vi "PHD2000 RUN SURE.vi"(8 "error in (no error)":errorcluster, 10 "Pump #":string, 11 "VISA resource name 2":refnum<visa-resource-name>) -> (0 "error out":errorcluster, 3 "VISA resource name out":refnum<visa-resource-name>)   [LabVIEW 2017]
uses:
  <instrlib>/Harvard Syringe Pump PHD2000/Harvard Syringe Pump PHD2000.lvlib
panel:
  out "Pump stop":bool
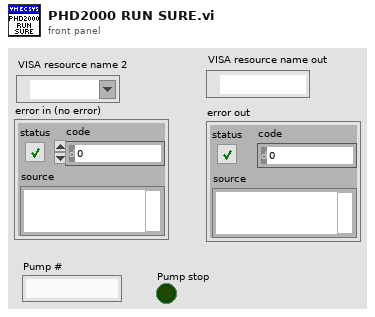
[diagram p1: front panel]
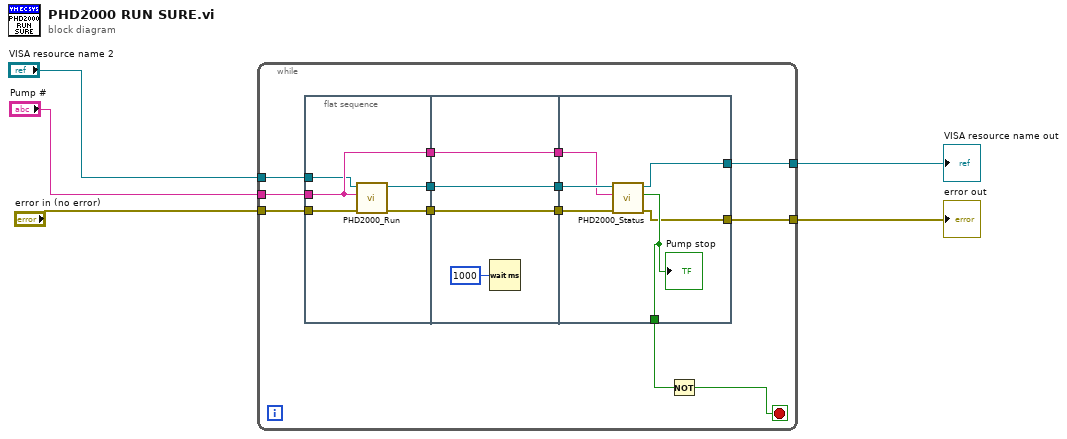
[diagram p0: block diagram]
diagram:
  n1 = while {
    tunnel: "Pump #" -> [w12]
    tunnel: "VISA resource name 2" -> [w11]
    tunnel: "error in (no error)" -> [w10]
    tunnel: [w7] -> w2
    tunnel: [w6] -> w1
    stop <- w9 stop-if-true
    n2 = flat-sequence {
      tunnel: w12 -> [w23]
      tunnel: [w23] -> w18
      tunnel: [w22] -> w17
      tunnel: w11 -> [w21]
      tunnel: [w20] -> w16
      tunnel: w10 -> [w19]
      tunnel: w18 -> [w27]
      tunnel: [w27] -> w15
      tunnel: w17 -> [w26]
      tunnel: [w26] -> w14
      tunnel: w16 -> [w25]
      tunnel: [w25] -> w13
      tunnel: w15 -> [w31]
      tunnel: w14 -> [w33]
      tunnel: w13 -> [w32]
      tunnel: [w30] -> w8
      tunnel: [w29] -> w7
      tunnel: [w28] -> w6
      frame #0 {
        n3 = call <instrlib>:"PHD2000_Run.vi"("VISA resource name 2"=w21, "Pump #"=w23, "error in (no error)"=w19) -> ("VISA resource name out"=w22:refnum<visa-resource-name>, "error out"=w20:errorcluster)  [unwired: 6 in]
      }
      frame #1 {
        n4 = Wait (ms)(milliseconds to wait=u32 1000) -> ()  [unwired: 1 out]
      }
      frame #2 {
        n5 = call <instrlib>:"PHD2000_Status.vi"("error in (no error)"=w32, "Pump #"=w31, "VISA resource name 2"=w33) -> ("error out"=w28:errorcluster, "Pump stop"=w30:bool, "VISA resource name out"=w29:refnum<visa-resource-name>)  [unwired: 3 in, 3 out]
        "Pump stop" <- w30
      }
    }
    n6 = Not(x=w8) -> (.not. x?=w9:bool)
  }
  "error out" <- w1
  "VISA resource name out" <- w2
